vi "ReadRegister.vi"(7 "I2C Connection":refnum<class "I2C Connection.lvclass">, 8 "error in (no error)":errorcluster, 10 "Register":T1) -> (0 "error out":errorcluster, 2 "Numeric":i16)   [LabVIEW 2020, in "CTI-Peripheral.lvlib" / "Grove 6 Axis Gyro Accel LSM6DS3.lvclass"]
uses:
  Grove 6 Axis Gyro Accel LSM6DS3.lvclass
  Register.ctl
  CTI/I2C Connection/I2C Connection.lvclass
  CTI/I2C Connection/I2C Connection.lvclass/I2C Connection.ctl
  CTI/Session/I2C Write Data.vi
  CTI/Session/I2C Read Data.vi
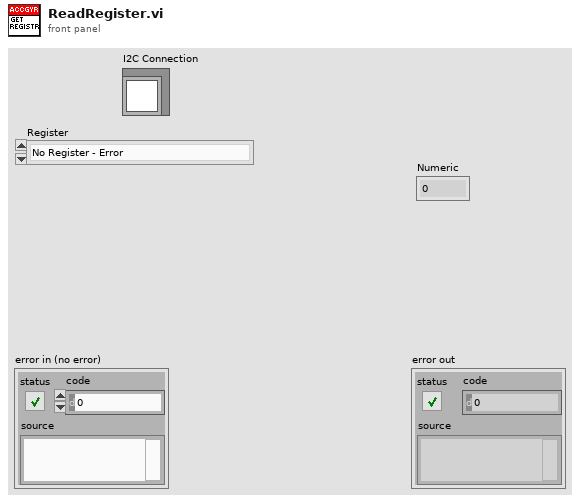
[diagram p1: front panel]
types:
  T1 = typedef "CTI-Peripheral.lvlib/Grove 6 Axis Gyro Accel LSM6DS3.lvclass/Register.ctl" = enum16{"No Register - Error", "D6D_SRC", "STATUS_REG", "OUT_TEMP_L", "OUT_TEMP_H", "OUTX_L_G", "OUTX_H_G", "OUTY_L_G", "OUTY_H_G", "OUTZ_L_G", "OUTZ_H_G", "OUTX_L_XL", "OUTX_H_XL", "OUTY_L_XL", "OUTY_H_XL", "OUTZ_L_XL", "OUTZ_H_XL", "SENSORHUB1_REG", "SENSORHUB2_REG", "SENSORHUB3_REG", "SENSORHUB4_REG", "SENSORHUB5_REG", "SENSORHUB6_REG", "SENSORHUB7_REG", "SENSORHUB8_REG", "SENSORHUB9_REG", "SENSORHUB10_REG", "SENSORHUB11_REG", "SENSORHUB12_REG"}
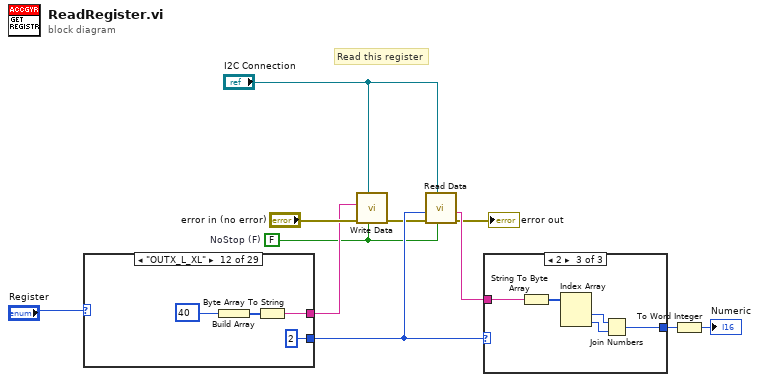
[diagram p0: block diagram]
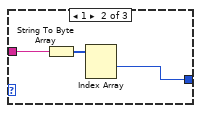
[diagram p3: hidden frame]
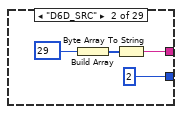
[diagram p5: hidden frame]
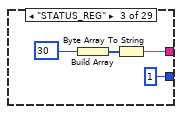
[diagram p6: hidden frame]
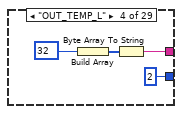
[diagram p7: hidden frame]
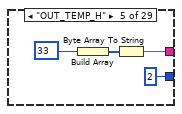
[diagram p8: hidden frame]
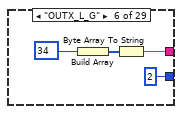
[diagram p9: hidden frame]
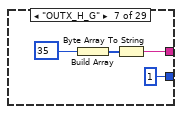
[diagram p10: hidden frame]
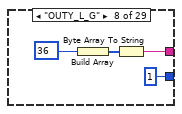
[diagram p11: hidden frame]
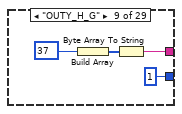
[diagram p12: hidden frame]
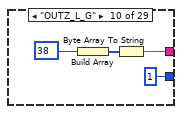
[diagram p13: hidden frame]
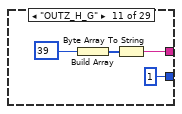
[diagram p14: hidden frame]
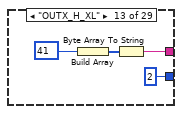
[diagram p15: hidden frame]
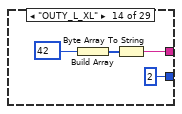
[diagram p16: hidden frame]
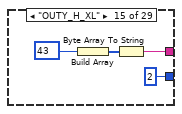
[diagram p17: hidden frame]
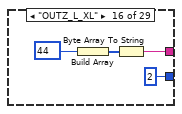
[diagram p18: hidden frame]
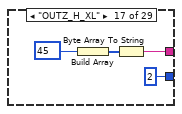
[diagram p19: hidden frame]
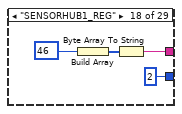
[diagram p20: hidden frame]
diagram:
  w2 = FALSE  # NoStop (F)
  # "Read this register"
  n1 = case shown="\"OUTX_L_XL\"" "Register" {
    tunnel: [_ w15 w19 w23 w27 w31 w35 w39 w43 w47 w51 w55 w59 w63 w67 w71 w75 w79 w83 w87 w91 w95 w99 w103 w107 w111 w115 w119 w123] -> w7
    tunnel: [_ u8 2 ("Len") u8 1 ("Len") u8 2 ("Len") u8 2 ("Len") u8 2 ("Len") u8 1 ("Len") u8 1 ("Len") u8 1 ("Len") u8 1 ("Len") u8 1 ("Len") u8 2 ("Len") u8 2 ("Len") u8 2 ("Len") u8 2 ("Len") u8 2 ("Len") u8 2 ("Len") u8 2 ("Len") u8 2 ("Len") u8 1 ("Len") u8 1 ("Len") u8 1 ("Len") u8 1 ("Len") u8 1 ("Len") u8 1 ("Len") u8 1 ("Len") u8 1 ("Len") u8 1 ("Len") u8 1 ("Len")] -> w6
    frame "No Register - Error", Default {
    }
    frame "D6D_SRC" {
      n2 = Build Array(u8 29 ("GYRO_OUTX_L_G")) -> (w13:u8[])
      n3 = Byte Array To String(unsigned byte array=w13) -> (string=w15:string)
    }
    frame "STATUS_REG" {
      n4 = Build Array(u8 30 ("GYRO_OUTX_L_G")) -> (w17:u8[])
      n5 = Byte Array To String(unsigned byte array=w17) -> (string=w19:string)
    }
    frame "OUT_TEMP_L" {
      n6 = Build Array(u8 32 ("GYRO_OUTX_L_G")) -> (w21:u8[])
      n7 = Byte Array To String(unsigned byte array=w21) -> (string=w23:string)
    }
    frame "OUT_TEMP_H" {
      n8 = Build Array(u8 33 ("GYRO_OUTX_L_G")) -> (w25:u8[])
      n9 = Byte Array To String(unsigned byte array=w25) -> (string=w27:string)
    }
    frame "OUTX_L_G" {
      n10 = Build Array(u8 34 ("GYRO_OUTX_L_G")) -> (w29:u8[])
      n11 = Byte Array To String(unsigned byte array=w29) -> (string=w31:string)
    }
    frame "OUTX_H_G" {
      n12 = Build Array(u8 35 ("GYRO_OUTX_L_G")) -> (w33:u8[])
      n13 = Byte Array To String(unsigned byte array=w33) -> (string=w35:string)
    }
    frame "OUTY_L_G" {
      n14 = Build Array(u8 36 ("GYRO_OUTX_L_G")) -> (w37:u8[])
      n15 = Byte Array To String(unsigned byte array=w37) -> (string=w39:string)
    }
    frame "OUTY_H_G" {
      n16 = Build Array(u8 37 ("GYRO_OUTX_L_G")) -> (w41:u8[])
      n17 = Byte Array To String(unsigned byte array=w41) -> (string=w43:string)
    }
    frame "OUTZ_L_G" {
      n18 = Build Array(u8 38 ("GYRO_OUTX_L_G")) -> (w45:u8[])
      n19 = Byte Array To String(unsigned byte array=w45) -> (string=w47:string)
    }
    frame "OUTZ_H_G" {
      n20 = Build Array(u8 39 ("GYRO_OUTX_L_G")) -> (w49:u8[])
      n21 = Byte Array To String(unsigned byte array=w49) -> (string=w51:string)
    }
    frame "OUTX_L_XL" {
      n22 = Build Array(u8 40 ("GYRO_OUTX_L_G")) -> (w53:u8[])
      n23 = Byte Array To String(unsigned byte array=w53) -> (string=w55:string)
    }
    frame "OUTX_H_XL" {
      n24 = Build Array(u8 41 ("GYRO_OUTX_L_G")) -> (w57:u8[])
      n25 = Byte Array To String(unsigned byte array=w57) -> (string=w59:string)
    }
    frame "OUTY_L_XL" {
      n26 = Build Array(u8 42 ("GYRO_OUTX_L_G")) -> (w61:u8[])
      n27 = Byte Array To String(unsigned byte array=w61) -> (string=w63:string)
    }
    frame "OUTY_H_XL" {
      n28 = Build Array(u8 43 ("GYRO_OUTX_L_G")) -> (w65:u8[])
      n29 = Byte Array To String(unsigned byte array=w65) -> (string=w67:string)
    }
    frame "OUTZ_L_XL" {
      n30 = Build Array(u8 44 ("GYRO_OUTX_L_G")) -> (w69:u8[])
      n31 = Byte Array To String(unsigned byte array=w69) -> (string=w71:string)
    }
    frame "OUTZ_H_XL" {
      n32 = Build Array(u8 45 ("GYRO_OUTX_L_G")) -> (w73:u8[])
      n33 = Byte Array To String(unsigned byte array=w73) -> (string=w75:string)
    }
    frame "SENSORHUB1_REG" {
      n34 = Build Array(u8 46 ("GYRO_OUTX_L_G")) -> (w77:u8[])
      n35 = Byte Array To String(unsigned byte array=w77) -> (string=w79:string)
    }
    frame "SENSORHUB2_REG" {
      n36 = Build Array(u8 47 ("GYRO_OUTX_L_G")) -> (w81:u8[])
      n37 = Byte Array To String(unsigned byte array=w81) -> (string=w83:string)
    }
    frame "SENSORHUB3_REG" {
      n38 = Build Array(u8 48 ("GYRO_OUTX_L_G")) -> (w85:u8[])
      n39 = Byte Array To String(unsigned byte array=w85) -> (string=w87:string)
    }
    frame "SENSORHUB4_REG" {
      n40 = Build Array(u8 49 ("GYRO_OUTX_L_G")) -> (w89:u8[])
      n41 = Byte Array To String(unsigned byte array=w89) -> (string=w91:string)
    }
    frame "SENSORHUB5_REG" {
      n42 = Build Array(u8 50 ("GYRO_OUTX_L_G")) -> (w93:u8[])
      n43 = Byte Array To String(unsigned byte array=w93) -> (string=w95:string)
    }
    frame "SENSORHUB6_REG" {
      n44 = Build Array(u8 51 ("GYRO_OUTX_L_G")) -> (w97:u8[])
      n45 = Byte Array To String(unsigned byte array=w97) -> (string=w99:string)
    }
    frame "SENSORHUB7_REG" {
      n46 = Build Array(u8 52 ("GYRO_OUTX_L_G")) -> (w101:u8[])
      n47 = Byte Array To String(unsigned byte array=w101) -> (string=w103:string)
    }
    frame "SENSORHUB8_REG" {
      n48 = Build Array(u8 53 ("GYRO_OUTX_L_G")) -> (w105:u8[])
      n49 = Byte Array To String(unsigned byte array=w105) -> (string=w107:string)
    }
    frame "SENSORHUB9_REG" {
      n50 = Build Array(u8 54 ("GYRO_OUTX_L_G")) -> (w109:u8[])
      n51 = Byte Array To String(unsigned byte array=w109) -> (string=w111:string)
    }
    frame "SENSORHUB10_REG" {
      n52 = Build Array(u8 55 ("GYRO_OUTX_L_G")) -> (w113:u8[])
      n53 = Byte Array To String(unsigned byte array=w113) -> (string=w115:string)
    }
    frame "SENSORHUB11_REG" {
      n54 = Build Array(u8 56 ("GYRO_OUTX_L_G")) -> (w117:u8[])
      n55 = Byte Array To String(unsigned byte array=w117) -> (string=w119:string)
    }
    frame "SENSORHUB12_REG" {
      n56 = Build Array(u8 57 ("GYRO_OUTX_L_G")) -> (w121:u8[])
      n57 = Byte Array To String(unsigned byte array=w121) -> (string=w123:string)
    }
  }
  n58 = call "Write Data.vi"("NoStop (F)"=w2, "I2C Connection"="I2C Connection", "error in (no error)"="error in (no error)", "Data"=w7) -> ("error out"=w4:errorcluster)  [unwired: 7 in]
  n59 = call "Read Data.vi"("NoStop (F)"=w2, "I2C Connection"="I2C Connection", "error in (no error)"=w4, "Len"=w6) -> ("error out"=→"error out":errorcluster, "Data"=w5:string)  [unwired: 6 in]
  n60 = case shown="2" w6 {
    tunnel: [_ w124 w131] -> w11
    tunnel: w5 -> [_ w125 w129]
    frame 0, Default {
    }
    frame 1 {
      n61 = String To Byte Array(string=w125) -> (unsigned byte array=w126:u8[])
      n62 = Index Array(array=w126) -> (element #1=w124:u8)  [unwired: 2 in, 1 out]
    }
    frame 2 {
      n63 = String To Byte Array(string=w129) -> (unsigned byte array=w130:u8[])
      n64 = Index Array(array=w130) -> (element #1=w128:u8, element #2=w127:u8)  [unwired: 2 in]
      n65 = Join Numbers(hi=w128, lo=w127) -> ((hi.lo)=w131:u16)
    }
  }
  n66 = To Word Integer(number=w11) -> (16bit integer=→"Numeric":i16)
